vi "Transform.vi"(8 "error in (no error)":errorcluster caption="entrée d'erreur (pas d'erreur)", 9 "y":string[][](array[string]), 10 "X":string[][](array[string]), 11 "FeatureHasher.lvclass":refnum<class "FeatureHasher.lvclass">) -> (0 "error out":errorcluster caption="sortie d'erreur", 2 "Data":T1, 3 "FeatureHasher.lvclass":refnum<class "FeatureHasher.lvclass">)   [LabVIEW 2020, in "FeatureHasher.lvclass"]
doc: "Transform a sequence of instances to a scipy.sparse matrix.\n\nReturns : \n\n- X : sparse matrix of shape (n_samples, n_features)\nFeature matrix, for use with estimators or further transformers."
uses:
  FeatureHasher.lvclass
  FeatureHasher.lvclass/FeatureHasher.ctl
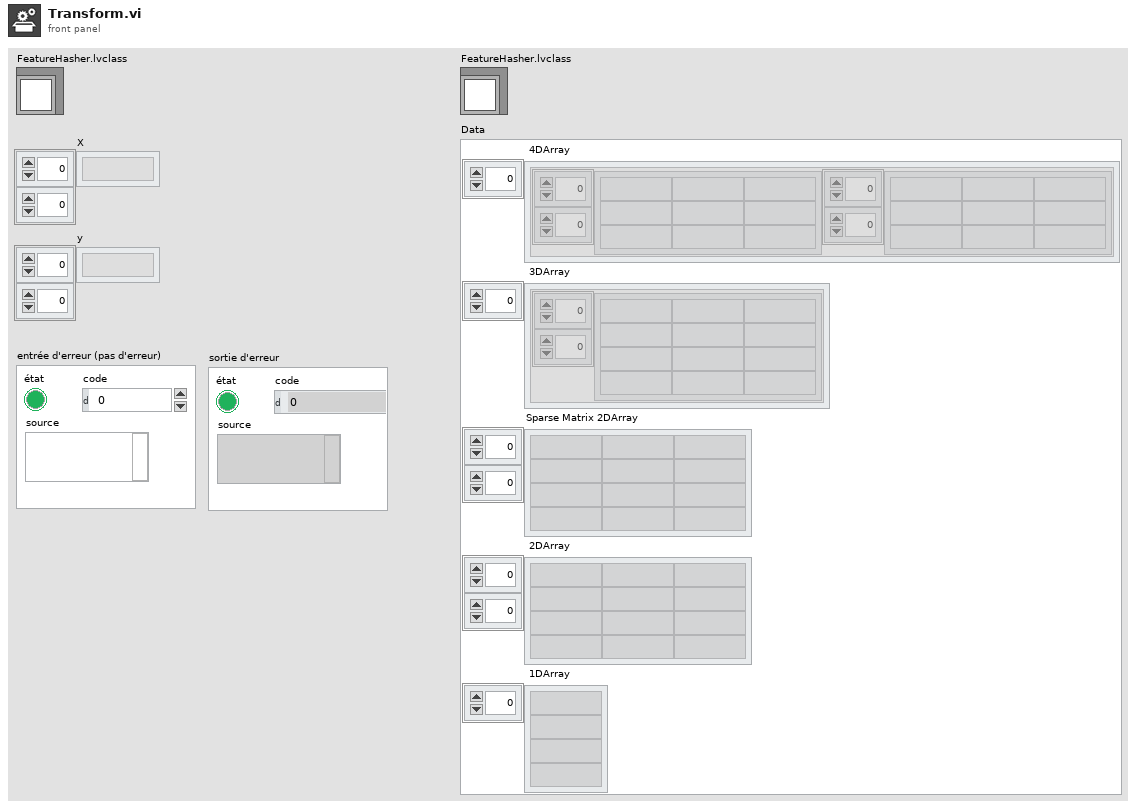
[diagram p1: front panel]
types:
  T1 = cluster{" 4DArray":cluster{"1":string[][], "2":string[][]}[], " 3DArray":cluster{"Tableau":string[][]}[], "Sparse Matrix 2DArray":string[][], " 2DArray":string[][], " 1DArray":string[]}
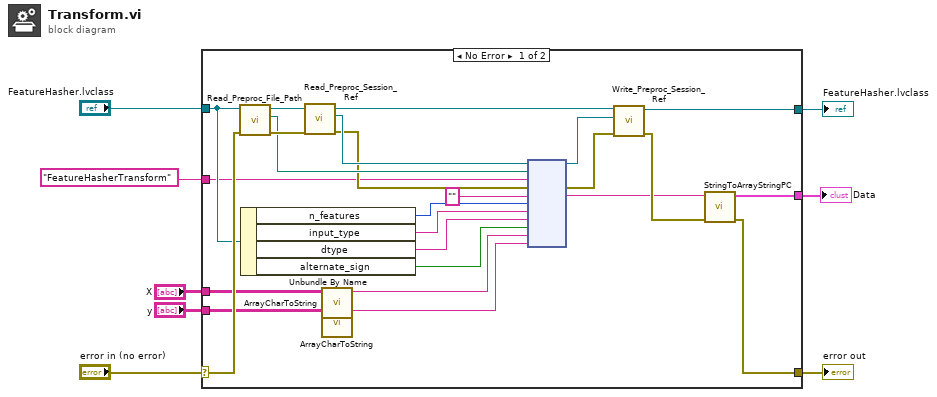
[diagram p0: block diagram]
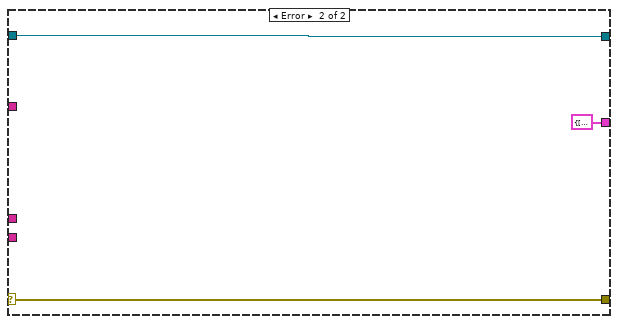
[diagram p2: hidden frame]
diagram:
  n1 = case shown="No Error" "error in (no error)" {
    selector: "error in (no error)" -> [w21 w36]
    tunnel: [w10 w36] -> w7
    tunnel: [w17 w35] -> w5
    tunnel: "FeatureHasher.lvclass" -> [w20 w35]
    tunnel: "FeatureHasherTransform" ("Fonction") -> [w19 _]
    tunnel: "X" -> [w16 _]
    tunnel: "y" -> [w15 _]
    tunnel: [w9 T1 {" 4DArray"=[], " 3DArray"=[], "Sparse Matrix 2DArray"=[], " 2DArray"=[], " 1DArray"=[]} ("Data")] -> w1
    frame No Error {
      n2 = call-dynamic "Read_Preproc_File_Path.vi"("error in (no error)"=w21, "Python in"=w20) -> ("error out"=w32:errorcluster, "File_Path"=w31:path, "Python out"=w33:refnum<class "FeatureHasher.lvclass">)  [unwired: 7 in]
      n3 = Unbundle By Name(w20) -> ("n_features"=w24:i32, "input_type"=w23:string, "dtype"=w22:string, "alternate_sign"=w18:bool)
      n4 = call-dynamic "Read_Preproc_Session_Ref.vi"("error in (no error)"=w32, "Python in"=w33) -> ("error out"=w29:errorcluster, "Session_ref"=w30:refnum<k35>, "Python out"=w28:refnum<class "FeatureHasher.lvclass">)  [unwired: 7 in]
      n5 = call "ArrayCharToString.vi"("TAB"=w16) -> ("Instruction"=w14:string)  [unwired: 10 in]
      n6 = call "ArrayCharToString.vi"("TAB"=w15) -> ("Instruction"=w13:string)  [unwired: 10 in]
      n7 = node(w30, w31, w19, w29, "", w24, w23, w22, w18, w14, w13) -> (w26:refnum<k35>, w27:errorcluster, w11:string)  [unwired: 6 in, 2 out]
      n8 = call-dynamic "Write_Preproc_Session_Ref.vi"("error in (no error)"=w27, "Session_ref"=w26, "Python in"=w28) -> ("error out"=w12:errorcluster, "Python out"=w17:refnum<class "FeatureHasher.lvclass">)  [unwired: 7 in]
      n9 = call "StringToArrayStringPC.vi"("sortie d'erreur"=w12, "Return value"=w11) -> ("sortie d'erreur"=w10:errorcluster, "Data"=w9:T1)  [unwired: 8 in]
    }
    frame Error {
    }
  }
  "error out" <- w7
  "FeatureHasher.lvclass" <- w5
  "Data" <- w1
